vi "Send Packet.vi"(6 "deadline":T1={"mode"=enum."Relative", "deadline (ms)"=30000}, 7 "priority":bool, 8 "error in":errorcluster, 10 "packet":T3 {"payload" format="%02x"}, 11 "connection in":refnum<class "Low Level Connection.lvclass">) -> (0 "error out":errorcluster, 2 "request id":u32, 3 "connection out":refnum<class "Low Level Connection.lvclass">)   [LabVIEW 2020, in "NI_SFTP.lvlib" / "Low Level Connection.lvclass"]
uses:
  <vilib>/net/SFTP/Low Level Connection/Low Level Connection.lvclass
  <vilib>/net/SFTP/Low Level Connection/Packet.ctl
  <vilib>/net/SFTP/Low Level Connection/Packet Type.ctl
  <vilib>/Utility/Deadline/Deadline.ctl
  <vilib>/Utility/Deadline/Mode.ctl
  <vilib>/net/SFTP/Low Level Connection/Low Level Connection.lvclass/Low Level Connection.ctl
  <vilib>/Array/Bytestream/Bytestream.lvclass/Bytestream.ctl
  6246e9f0-63c2-3fec-0064-7420e449d63f.vi
  c3f8dbf6-1016-3fe8-001d-0e448bfa933f.vi
  7312759c-d8b4-3fd7-9a13-c6a052c2ec3f.vi
  6246e9f0-63c2-3fec-0064-7420e449d63f.vi/bdc7a191-7bf0-4445-83d9-77b7daf5808b.vi
  c3f8dbf6-1016-3fe8-001d-0e448bfa933f.vi/2c32e142-d777-4ea3-96d3-1b889caf94bd.vi
  <vilib>/Array/Bytestream/Append.vi
  <vilib>/Array/Bytestream/Grow If Necessary.vi
  <vilib>/Array/Bytestream/Next Available Datum Index.vi
  <vilib>/Array/Bytestream/Count Allocated Datums.vi
  <vilib>/Array/Bytestream/Count Datums.vi
  <vilib>/Array/Bytestream/Grow Datum Array.vi
  <vilib>/Utility/error.llb/Error Cluster From Error Code.vi
  <vilib>/Array/Bytestream/Bytestream.lvclass
  <vilib>/ErrorRing/Error Ring.xnode
  <vilib>/Utility/Deadline/NI_Deadline.lvlib
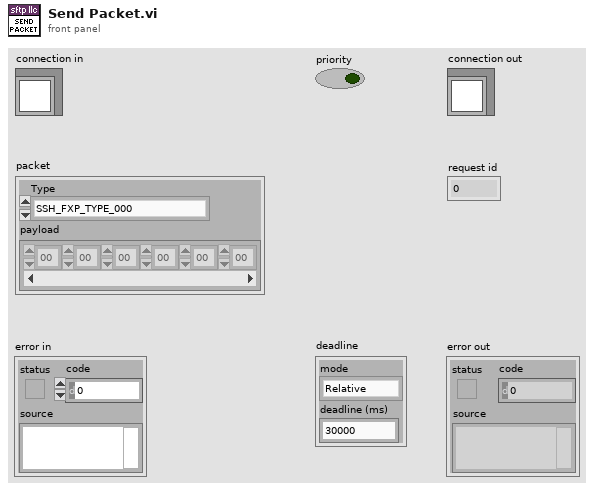
[diagram p1: front panel]
types:
  T1 = typedef "NI_Deadline.lvlib/Deadline.ctl" = cluster{"mode":T2, "deadline (ms)":u32}
  T2 = typedef "NI_Deadline.lvlib/Mode.ctl" = enum16{"Relative", "Use deadline", "Wait forever", "Nonblocking", "N/A"}
  T3 = typedef "NI_SFTP.lvlib/Low Level Connection.lvclass/Packet.ctl" = cluster{"Type":T4, "payload":u8[]}
  T4 = typedef "NI_SFTP.lvlib/Low Level Connection.lvclass/Packet Type.ctl" = enum16{"SSH_FXP_TYPE_000", "SSH_FXP_INIT", "SSH_FXP_VERSION", "SSH_FXP_OPEN", "SSH_FXP_CLOSE", "SSH_FXP_READ", "SSH_FXP_WRITE", "SSH_FXP_LSTAT", "SSH_FXP_FSTAT", "SSH_FXP_SETSTAT", "SSH_FXP_FSETSTAT", "SSH_FXP_OPENDIR", "SSH_FXP_READDIR", "SSH_FXP_REMOVE", "SSH_FXP_MKDIR", "SSH_FXP_RMDIR", "SSH_FXP_REALPATH", "SSH_FXP_STAT", "SSH_FXP_RENAME", "SSH_FXP_READLINK", "SSH_FXP_SYMLINK", "SSH_FXP_LINK", "SSH_FXP_BLOCK", "SSH_FXP_UNBLOCK", "SSH_FXP_TYPE_024", "SSH_FXP_TYPE_025", "SSH_FXP_TYPE_026", "SSH_FXP_TYPE_027", "SSH_FXP_TYPE_028", "SSH_FXP_TYPE_029", "SSH_FXP_TYPE_030", "SSH_FXP_TYPE_031", "SSH_FXP_TYPE_032", "SSH_FXP_TYPE_033", "SSH_FXP_TYPE_034", "SSH_FXP_TYPE_035", "SSH_FXP_TYPE_036", "SSH_FXP_TYPE_037", "SSH_FXP_TYPE_038", "SSH_FXP_TYPE_039", "SSH_FXP_TYPE_040", "SSH_FXP_TYPE_041", "SSH_FXP_TYPE_042", "SSH_FXP_TYPE_043", "SSH_FXP_TYPE_044", "SSH_FXP_TYPE_045", "SSH_FXP_TYPE_046", "SSH_FXP_TYPE_047", "SSH_FXP_TYPE_048", "SSH_FXP_TYPE_049", "SSH_FXP_TYPE_050", "SSH_FXP_TYPE_051", "SSH_FXP_TYPE_052", "SSH_FXP_TYPE_053", "SSH_FXP_TYPE_054", "SSH_FXP_TYPE_055", "SSH_FXP_TYPE_056", "SSH_FXP_TYPE_057", "SSH_FXP_TYPE_058", "SSH_FXP_TYPE_059", "SSH_FXP_TYPE_060", "SSH_FXP_TYPE_061", "SSH_FXP_TYPE_062", "SSH_FXP_TYPE_063", "SSH_FXP_TYPE_064", "SSH_FXP_TYPE_065", "SSH_FXP_TYPE_066", "SSH_FXP_TYPE_067", "SSH_FXP_TYPE_068", "SSH_FXP_TYPE_069", "SSH_FXP_TYPE_070", "SSH_FXP_TYPE_071", "SSH_FXP_TYPE_072", "SSH_FXP_TYPE_073", "SSH_FXP_TYPE_074", "SSH_FXP_TYPE_075", "SSH_FXP_TYPE_076", "SSH_FXP_TYPE_077", "SSH_FXP_TYPE_078", "SSH_FXP_TYPE_079", "SSH_FXP_TYPE_080", "SSH_FXP_TYPE_081", "SSH_FXP_TYPE_082", "SSH_FXP_TYPE_083", "SSH_FXP_TYPE_084", "SSH_FXP_TYPE_085", "SSH_FXP_TYPE_086", "SSH_FXP_TYPE_087", "SSH_FXP_TYPE_088", "SSH_FXP_TYPE_089", "SSH_FXP_TYPE_090", "SSH_FXP_TYPE_091", "SSH_FXP_TYPE_092", "SSH_FXP_TYPE_093", "SSH_FXP_TYPE_094", "SSH_FXP_TYPE_095", "SSH_FXP_TYPE_096", "SSH_FXP_TYPE_097", "SSH_FXP_TYPE_098", "SSH_FXP_TYPE_099", "SSH_FXP_TYPE_100", "SSH_FXP_STATUS", "SSH_FXP_HANDLE", "SSH_FXP_DATA", "SSH_FXP_NAME", "SSH_FXP_ATTRS", "SSH_FXP_TYPE_106", "SSH_FXP_TYPE_107", "SSH_FXP_TYPE_108", "SSH_FXP_TYPE_109", "SSH_FXP_TYPE_110", "SSH_FXP_TYPE_111", "SSH_FXP_TYPE_112", "SSH_FXP_TYPE_113", "SSH_FXP_TYPE_114", "SSH_FXP_TYPE_115", "SSH_FXP_TYPE_116", "SSH_FXP_TYPE_117", "SSH_FXP_TYPE_118", "SSH_FXP_TYPE_119", "SSH_FXP_TYPE_120", "SSH_FXP_TYPE_121", "SSH_FXP_TYPE_122", "SSH_FXP_TYPE_123", "SSH_FXP_TYPE_124", "SSH_FXP_TYPE_125", "SSH_FXP_TYPE_126", "SSH_FXP_TYPE_127", "SSH_FXP_TYPE_128", "SSH_FXP_TYPE_129", "SSH_FXP_TYPE_130", "SSH_FXP_TYPE_131", "SSH_FXP_TYPE_132", "SSH_FXP_TYPE_133", "SSH_FXP_TYPE_134", "SSH_FXP_TYPE_135", "SSH_FXP_TYPE_136", "SSH_FXP_TYPE_137", "SSH_FXP_TYPE_138", "SSH_FXP_TYPE_139", "SSH_FXP_TYPE_140", "SSH_FXP_TYPE_141", "SSH_FXP_TYPE_142", "SSH_FXP_TYPE_143", "SSH_FXP_TYPE_144", "SSH_FXP_TYPE_145", "SSH_FXP_TYPE_146", "SSH_FXP_TYPE_147", "SSH_FXP_TYPE_148", "SSH_FXP_TYPE_149", "SSH_FXP_TYPE_150", "SSH_FXP_TYPE_151", "SSH_FXP_TYPE_152", "SSH_FXP_TYPE_153", "SSH_FXP_TYPE_154", "SSH_FXP_TYPE_155", "SSH_FXP_TYPE_156", "SSH_FXP_TYPE_157", "SSH_FXP_TYPE_158", "SSH_FXP_TYPE_159", "SSH_FXP_TYPE_160", "SSH_FXP_TYPE_161", "SSH_FXP_TYPE_162", "SSH_FXP_TYPE_163", "SSH_FXP_TYPE_164", "SSH_FXP_TYPE_165", "SSH_FXP_TYPE_166", "SSH_FXP_TYPE_167", "SSH_FXP_TYPE_168", "SSH_FXP_TYPE_169", "SSH_FXP_TYPE_170", "SSH_FXP_TYPE_171", "SSH_FXP_TYPE_172", "SSH_FXP_TYPE_173", "SSH_FXP_TYPE_174", "SSH_FXP_TYPE_175", "SSH_FXP_TYPE_176", "SSH_FXP_TYPE_177", "SSH_FXP_TYPE_178", "SSH_FXP_TYPE_179", "SSH_FXP_TYPE_180", "SSH_FXP_TYPE_181", "SSH_FXP_TYPE_182", "SSH_FXP_TYPE_183", "SSH_FXP_TYPE_184", "SSH_FXP_TYPE_185", "SSH_FXP_TYPE_186", "SSH_FXP_TYPE_187", "SSH_FXP_TYPE_188", "SSH_FXP_TYPE_189", "SSH_FXP_TYPE_190", "SSH_FXP_TYPE_191", "SSH_FXP_TYPE_192", "SSH_FXP_TYPE_193", "SSH_FXP_TYPE_194", "SSH_FXP_TYPE_195", "SSH_FXP_TYPE_196", "SSH_FXP_TYPE_197", "SSH_FXP_TYPE_198", "SSH_FXP_TYPE_199", "SSH_FXP_EXTENDED", "SSH_FXP_EXTENDED_REPLY"}
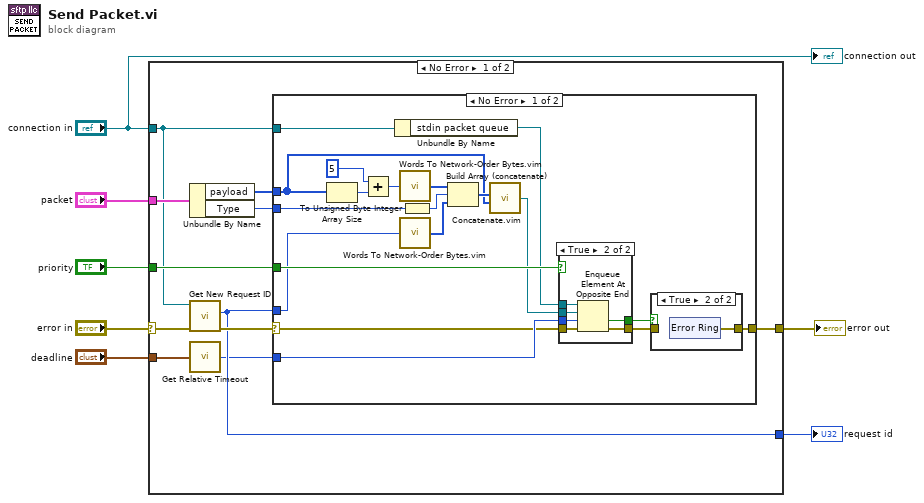
[diagram p0: block diagram]
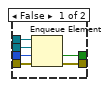
[diagram p3: hidden frame]
diagram:
  n1 = case shown="No Error" "error in" {
    selector: "error in" -> [w13 w57]
    tunnel: [w14 w57] -> w6
    tunnel: "connection in" -> [w10 _]
    tunnel: [w11 _] -> w5
    tunnel: "packet" -> [w17 _]
    tunnel: "priority" -> [w15 _]
    tunnel: "deadline" -> [w9 _]
    frame No Error {
      n2 = Unbundle By Name(w17) -> ("payload"=w16:u8[], "Type"=w18:T4)
      n3 = call <vilib>:"Get New Request ID.vi"("error in"=w13, "connection in"=w10) -> ("error out"=w12:errorcluster, "id"=w11:u32)  [unwired: 7 in, 1 out]
      n4 = call <vilib>:"Get Relative Timeout.vi"("Timeout"=w9) -> ("timeout (ms) out"=w8:i32)
      n5 = case shown="No Error" w12 {
        selector: w12 -> [w21 w56]
        tunnel: [w37 w56] -> w14
        tunnel: w18 -> [w35 _]
        tunnel: w16 -> [w28 _]
        tunnel: w15 -> [w27 _]
        tunnel: w8 -> [w22 _]
        tunnel: w11 -> [w20 _]
        tunnel: w10 -> [w19 _]
        frame No Error {
          n6 = Array Size(array=w28) -> (size(s)=w31:i32)
          n7 = Add(x=5, y=w31) -> (x+y=w32:i32)
          n8 = Unbundle By Name(w19) -> ("stdin packet queue"=w26:refnum<queue>)
          n9 = call "Words To Network-Order Bytes.vim"("word"=w32) -> ("bytes"=w33:u8[])
          n10 = call "Words To Network-Order Bytes.vim"("word"=w20) -> ("bytes"=w34:u8[])
          n11 = To Unsigned Byte Integer(number=w35) -> (unsigned 8bit integer=w36:u8)
          n12 = Build Array (concatenate)(w33, w36, w34) -> (w29:u8[])
          n13 = call "Concatenate.vim"("b"=w28, "a"=w29) -> ("a+b"=w25:refnum<class "Bytestream.lvclass">)  [unwired: 2 in]
          n14 = case shown="True" w27 {
            tunnel: w26 -> [w49 w55]
            tunnel: w25 -> [w46 w54]
            tunnel: w22 -> [w47 w53]
            tunnel: w21 -> [w48 w52]
            tunnel: [w45 w51] -> w24
            tunnel: [w44 w50] -> w23
            frame False {
              n15 = Enqueue Element(queue=w49, element=w46, timeout in ms (-1)=w47, error in (no error)=w48) -> (timed out?=w45:bool, error out=w44:errorcluster)  [unwired: 1 out]
            }
            frame True {
              n16 = Enqueue Element At Opposite End(queue=w55, element=w54, timeout in ms (-1)=w53, error in (no error)=w52) -> (timed out?=w51:bool, error out=w50:errorcluster)  [unwired: 1 out]
            }
          }
          n17 = case shown="True" w24 {
            tunnel: w23 -> [w38 _]
            tunnel: [w38 w39] -> w37
            frame False {
            }
            frame True {
              n18 = xnode "Error Ring"() -> ("error out"=w39:errorcluster)
            }
          }
        }
        frame Error {
        }
      }
    }
    frame Error {
    }
  }
  "error out" <- w6
  "request id" <- w5
  "connection out" <- "connection in"
